vi "Thevenin Source Calibration.vi"(11 "State":T2) -> ()   [LabVIEW 2015]
uses:
  Utility VIs/Type Defs/Speaker ring.ctl
  Cochlear Function Test Suite/LV Source/CFTS Main Panel SubVIs/CFTS-Experiment State.ctl
  Utility VIs/Controls/KListboxEx/KListboxEx.xctl
  Typedefs/Thev-State.ctl
  Typedefs/Thev-Procedure Phase.ctl
  Typedefs/Thev-Progress Table Element.ctl
  Typedefs/Thev-Optimization Result.ctl
  Typedefs/Thev-Parameters.ctl
  Typedefs/Thev-Stimulus.ctl
  Typedefs/Thev-Find.ctl
  Misc VIs/Equipment Control/ER10X/ER10X-Probe.ctl
  Typedefs/Thev-Optimization Parameters.ctl
  D:/Experiment VIs/Misc VIs/Equipment Control/ER10X/ER10XConnect.NET.dll
  Misc VIs/Equipment Control/ER10X/ER10XConnect.NET.dll
  Utility VIs/Conversion VIs/Create Waveform Cluster (2D).vi
  Utility VIs/Math VIs/FFT x(t) to dB,Degrees (2D).vi
panel:
  in  "Test":enum16{"Lengths", "Frequencies"}(ring)
  in  "Nulls":i32(xcontrol) caption="Null frequencies (Hz)"
  out "Probe B":bool
  out "Probe A":bool
  in  "Start":bool
  in  "Stop":bool
  in  "Find":T1={"precision"=10.0, "Nattempts"=6, "Navgs/att"=64} caption="Optimize positions"
  in  "Averages":i32=128
  in  "Speaker":T3
  in  "mic gain":dbl caption="Gain (dB)" min=0.0 max=40.0 step=1.0
  in  "Stimulus":T4={"Resolution (Hz)"=50.0, "Attenuation (dB)"=30.0, "Sampling rate (Hz)"=100000.0}
  out "Stimulus graph":cluster{i32, dbl, dbl[]}(graph)={0, 0.01, []}
  in  "Diameter":dbl=128.0 caption="Cavity diameter (cm)"
  in  "Compute":bool
  out "Log":string
  out "Progress":string[][](table)
  in  "Tabs":T5(tab)
  out "Mic signals":cluster{"offset":dbl, "dx":dbl, "Y":dbl[][]}(graph)
  out "Mic mag":cluster{"offset":dbl, "dx":dbl, "Y":dbl[][]}(graph)
  out "Acquired":i32=256
  out "Magnitude":cluster{"Frequency":dbl[], "Frequency":dbl[]}[](graph)
  out "Phase":cluster{"Frequency":dbl[], "Frequency":dbl[]}[](graph)
  out "Zx mag":cluster{"Frequency":dbl[], "Frequency":dbl[]}[](graph)
  out "Zx phase":cluster{"Frequency":dbl[], "Frequency":dbl[]}[](graph)
  out "Z0":cluster{"Frequency":dbl[], "Frequency":dbl[]}[](graph)
  out "P0":cluster{"Frequency":dbl[], "Frequency":dbl[]}[](graph)
  in  "result":cluster{"Path":path, "error ":errorcluster}
  out "Mic phase":cluster{"offset":dbl, "dx":dbl, "Y":dbl[][]}(graph)
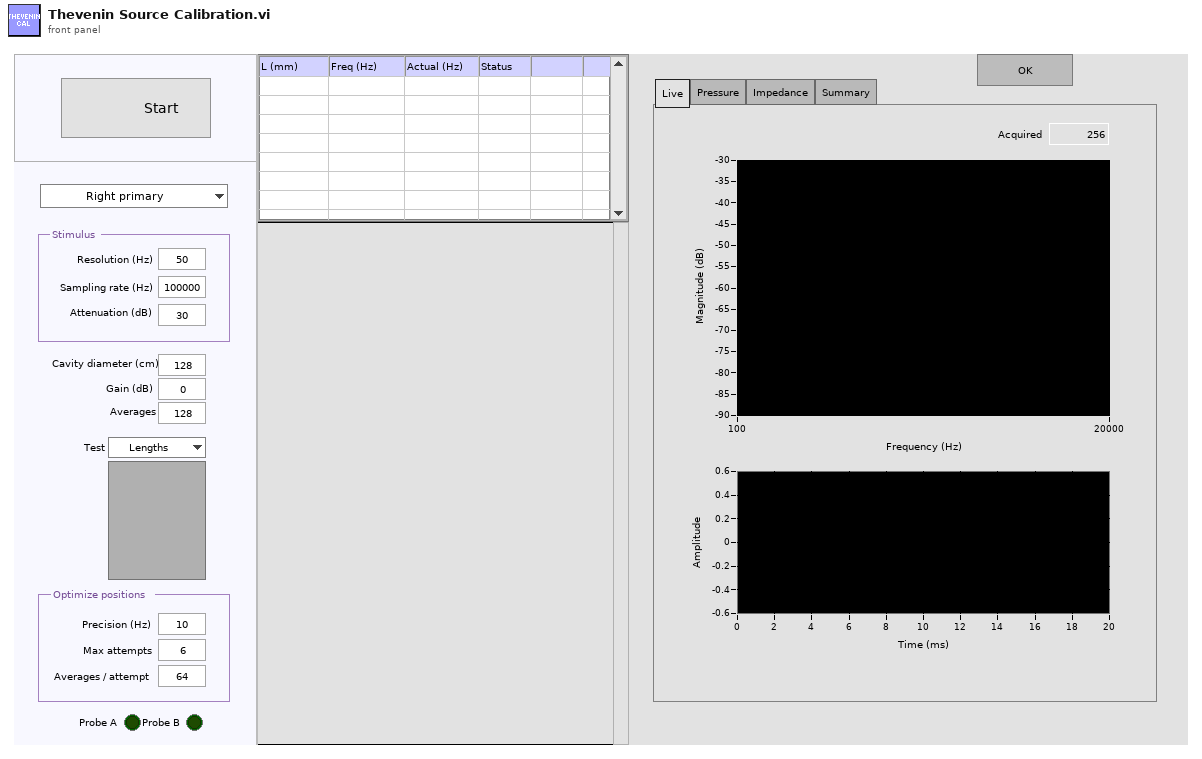
[diagram p1: front panel]
types:
  T1 = cluster{"precision":dbl, "Nattempts":i32, "Navgs/att":i32}
  T2 = typedef "CFTS-Experiment State.ctl" = cluster{"Experimenter":string, "Number":u32, "Right":string, "Left":string, "Data Folder":path, "State File":path, "Version Info":string, "End Exposure Time":dbl, "Exposure Duration":string, "Run #":cluster{"CAP":i16, "ABR":i16, "DP":i16, "VsEP":i16, "MeasSeq":i16, "SubSeq":i16, "SFOAE":i16}}
  T3 = typedef "Speaker ring.ctl" = enum16{"Right primary", "Right secondary", "Left primary", "Left secondary"}
  T4 = cluster{"Resolution (Hz)":dbl, "Attenuation (dB)":dbl, "Sampling rate (Hz)":dbl}
  T5 = enum32{"Live", "Pressure", "Impedance", "Summary"}
  T6 = typedef "Thev-Parameters.ctl" = cluster{"Speaker":enum16{"Right primary", "Right secondary", "Left primary", "Left secondary"}, "Chirp":T7, "Find":T8, "Gain (dB)":dbl, "Navgs":i32, "Diameter":dbl, "test points":dbl[], "Rprobe":T9, "LProbe":T9, "Mode":enum16{"Length", "Freq"}, "Optim":T10}
  T7 = typedef "Thev-Stimulus.ctl" = cluster{"resol (Hz)":dbl, "atten (dB)":dbl, "Fs (Hz)":dbl}
  T8 = typedef "Thev-Find.ctl" = cluster{"precision":dbl, "Nattempts":i32, "Navgs/att":i32}
  T9 = typedef "ER10X-Probe.ctl" = i32
  T10 = typedef "Thev-Optimization Parameters.ctl" = cluster{"Fmin":dbl, "Fmax":dbl}
  T11 = typedef "Thev-State.ctl" = cluster{"next":i32, "ER10X":refnum<k24>, "phase":T12, "progress":T13[], "folder":path, "log":string, "history":cluster{"L":dbl[], "F":dbl[]}, "optim":T14}
  T12 = typedef "Thev-Procedure Phase.ctl" = enum16{"Optimize", "Measure", "Compute", "Finished"}
  T13 = typedef "Thev-Progress Table Element.ctl" = cluster{"Freq":dbl, "Actual":dbl, "Pos":dbl, "Status":enum16{"None", "Measuring", "Finished"}, "Attempts":i32}
  T14 = typedef "Thev-Optimization Result.ctl" = cluster{"MSE":dbl, "Niter":i32, "Linit":dbl[], "Lfinal":dbl[]}
  T15 = typedef "KListboxEx.xctl/Events.ctl" = cluster{"Items Changed":refnum<user-event>, "List Changed":refnum<user-event>}
  T16 = enum16{"Right primary", "Right secondary", "Left primary", "Left secondary"}
  T17 = enum8{"Enabled", "Disabled", "Disabled and Grayed Out"}
  T18 = typedef "Cal Stimulus.ctl" = cluster{"Min Freq (Hz)":dbl, "Max Freq (Hz)":dbl, "Freq Step (Hz)":dbl, "Waveform":enum16{"Chirp", "Weighted"}, "Attenuation (dB)":dbl, "Sample Rate (Hz)":dbl}
  T19 = cluster{"new file path":path, "error out":errorcluster}
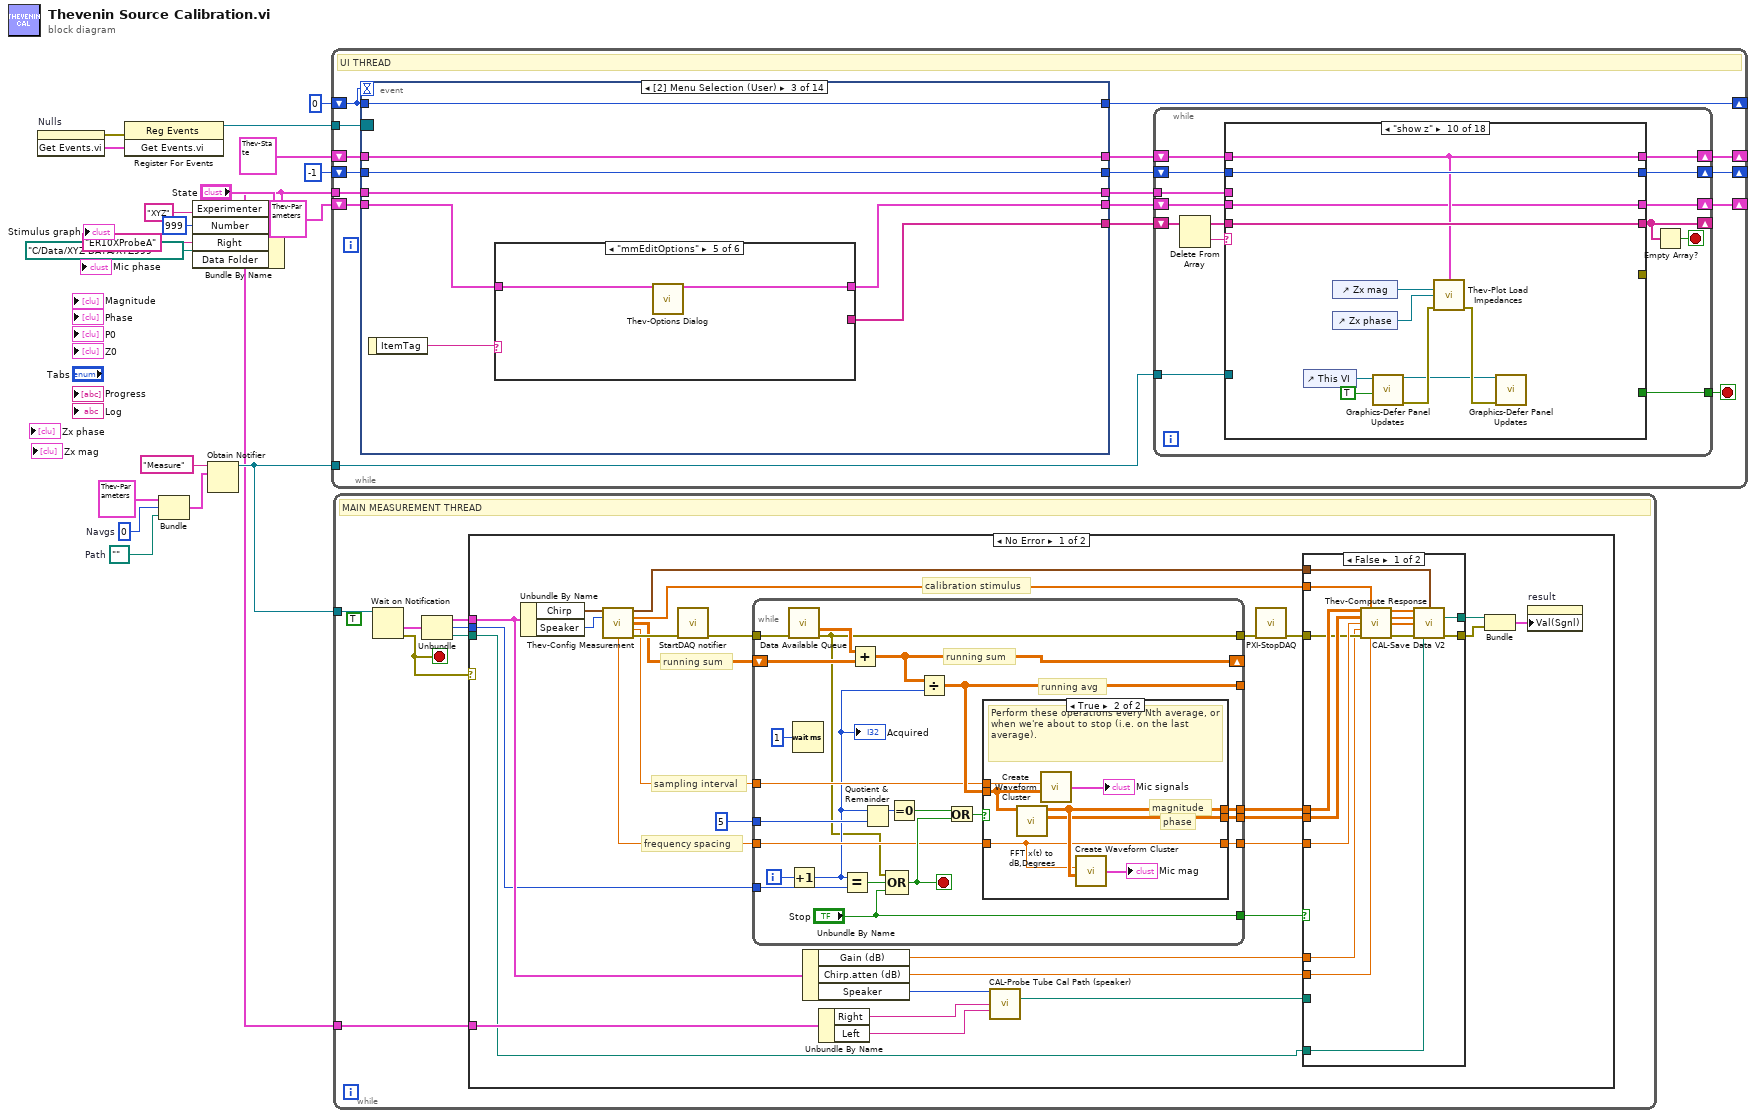
[diagram p0: block diagram]
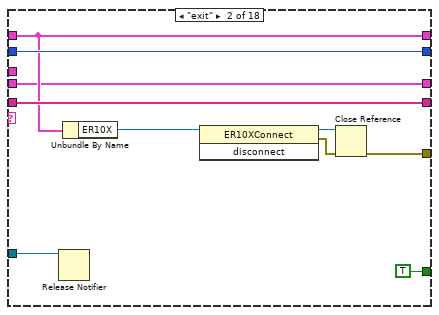
[diagram p6: hidden frame]
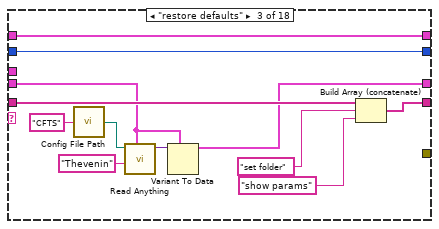
[diagram p7: hidden frame]
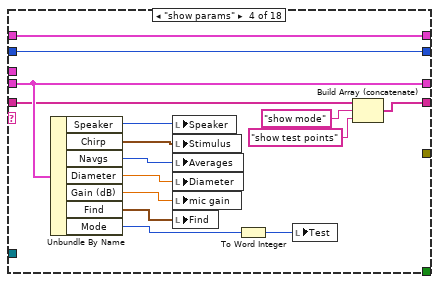
[diagram p8: hidden frame]
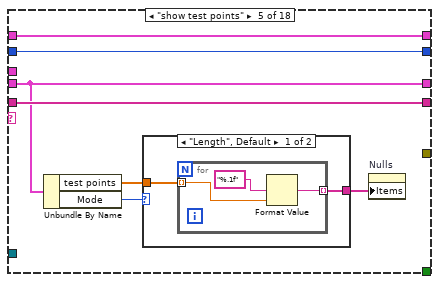
[diagram p9: hidden frame]
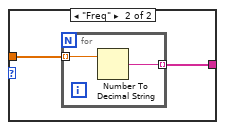
[diagram p10: hidden frame]
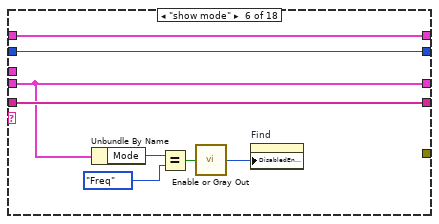
[diagram p11: hidden frame]
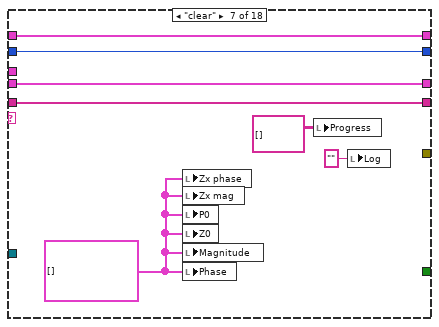
[diagram p12: hidden frame]
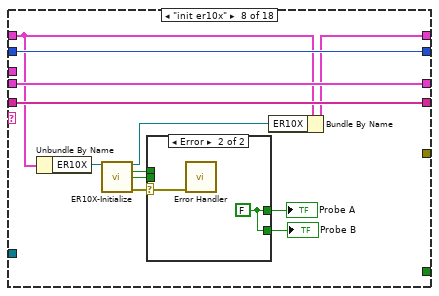
[diagram p13: hidden frame]
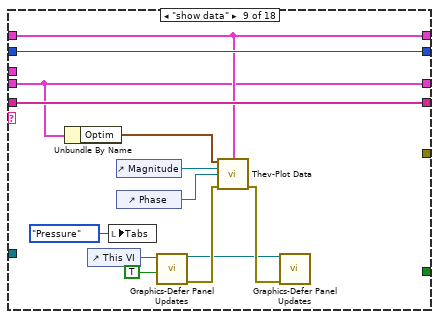
[diagram p15: hidden frame]
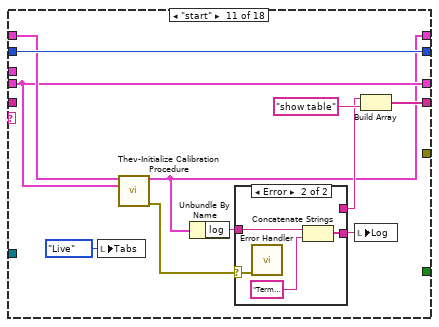
[diagram p16: hidden frame]
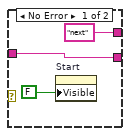
[diagram p17: hidden frame]
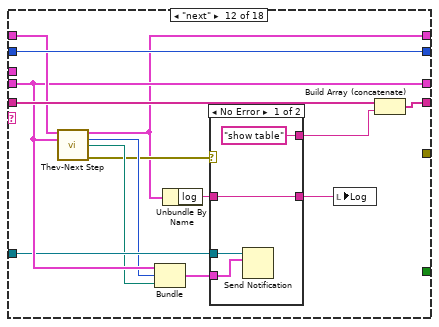
[diagram p18: hidden frame]
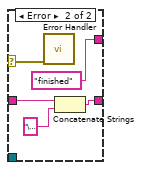
[diagram p19: hidden frame]
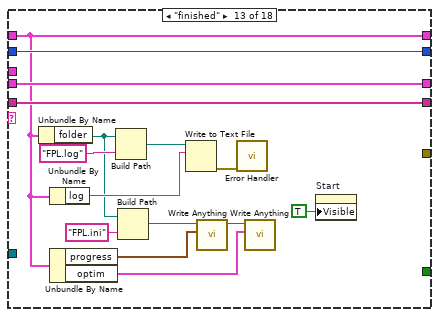
[diagram p20: hidden frame]
diagram:
  w10 = 0  # Navgs
  w9 = path ""  # Path
  n1 = invoke on="Nulls" class="KListboxEx (strict)" method="Get Events.vi"() -> (error out=w8:errorcluster, "Get Events.vi"=w7:T15)  [unwired: 3 in, 1 out]
  n2 = register-events(error in=w8, w7) -> (reference out=w6:refnum<event-registration>)  [unwired: 1 in, 1 out]
  n3 = Bundle("Params"=T6 {"Speaker"=enum."Right primary", "Chirp"={"resol (Hz)"=50.0, "atten (dB)"=20.0, "Fs (Hz)"=100000.0}, "Find"={"precision"=10.0, "Nattempts"=6, "Navgs/att"=64}, "Gain (dB)"=40.0, "Navgs"=128, "Diameter"=0.8, "test points"=[2878.0, 3289.0, 4112.0, 4638.0, 5345.0, 7401.0], "Rprobe"=0, "LProbe"=0, "Mode"=enum."Length", "Optim"={"Fmin"=0.0, "Fmax"=0.0}}, "Navgs"=w10, "Path"=w9) -> (w11:cluster{"Params":T6, "Navgs":i32, "Path":path})  [unwired: 1 in]
  n4 = Bundle By Name(cluster="State", "Experimenter"="XYZ", "Number"=u32 999, "Right"="ER10XProbeA", "Data Folder"=path "C:/Data/XYZ DATA/XYZ999") -> (w5:T2)
  n5 = Obtain Notifier(name (unnamed)="Measure", notification data type=w11) -> (notifier out=w19:refnum<notifier>)  [unwired: 2 in, 2 out]
  n6 = while {
    tunnel: w19 -> [w25]
    shift-right: [w34] -> _
    shift-left: 0 -> [w35]
    shift-right: [w28] -> _
    shift-left: -1 -> [w36]
    tunnel: w5 -> [w33]
    shift-right: [w29] -> _
    shift-left: T6 {"Speaker"=enum."Right primary", "Chirp"={"resol (Hz)"=50.0, "atten (dB)"=20.0, "Fs (Hz)"=100000.0}, "Find"={"precision"=10.0, "Nattempts"=6, "Navgs/att"=64}, "Gain (dB)"=40.0, "Navgs"=128, "Diameter"=0.8, "test points"=[2878.0, 3289.0, 4112.0, 4638.0, 5345.0, 7401.0], "Rprobe"=1, "LProbe"=0, "Mode"=enum."Freq", "Optim"={"Fmin"=500.0, "Fmax"=10000.0}} ("Params") -> [w32]
    shift-right: [w21] -> _
    shift-left: T11 {"next"=0, "ER10X"=refnum, "phase"=enum."Optimize", "progress"=[], "folder"=path "", "log"="", "history"={"L"=[], "F"=[]}, "optim"={"MSE"=0.0, "Niter"=0, "Linit"=[], "Lfinal"=[]}} -> [w23]
    tunnel: w6 -> [w20]
    stop <- w26 stop-if-true
    # "UI THREAD"
    n7 = event shown="[2] Menu Selection (User)" {
      selector: w20 -> [_ _ _ _ _ _ _ _ _ _ _ _ _ _]
      dyn-events: _ -> [_ _ _ _ _ _ _ _ _ _ _ _ _ _]
      timeout: w35 -> [_ _ _ _ _ _ _ _ _ _ _ _ _ _]
      tunnel: w36 -> [w313 w322 w331 w353 w368 w375 w382 w394 w401 w414 w443 w455 w467 w504]
      tunnel: [w313 w322 w331 w353 w368 w375 w382 w394 w401 w414 w443 w455 w467 w504] -> w31
      tunnel: w35 -> [_ w321 w330 w352 w367 w380 w387 w393 w400 w413 w442 w454 w466 w503]
      tunnel: [-1 w321 w330 w352 w367 w380 w387 w393 w400 w413 w442 w454 w466 w503] -> w34
      tunnel: w33 -> [w305 w318 w325 w351 w357 w378 w385 w390 w397 w412 w440 w451 w465 w501]
      tunnel: w32 -> [w303 w320 w328 w350 w366 w379 w386 w392 w399 w403 w441 w453 w461 w502]
      tunnel: [w303 w320 w327 w350 w365 w377 w384 w391 w398 w410 w438 w452 w461 w502] -> w30
      tunnel: [string[] ["init er10x", "restore defaults"] string[] ["exit"] w326 string[] ["start"] w354 _ _ _ _ string[] ["show mode", "show test points"] _ _ w459 string[] ["compute"]] -> w27
      tunnel: [w305 w318 w325 w351 w357 w378 w385 w390 w397 w412 w440 w451 w465 w501] -> w24
      tunnel: w23 -> [w302 w317 w324 w349 w356 w374 w381 w388 w396 w411 w439 w450 w462 w500]
      tunnel: [w302 w317 w324 w349 w355 w374 w381 w388 w396 w411 w439 w450 w457 w500] -> w22
      event Timeout {
        n8 = event-data() -> ()  [unwired: 1 in, 1 out]
        n9 = property on="Nulls" class="KListboxEx (strict)"() -> ("Ref"=w310:refnum<vi>)  [unwired: 2 in, 2 out]
        n10 = property class="LstBox (strict)"(reference=w310, "Horizontal Lines Visible"=TRUE ("Visible Items:Horizontal Lines Visible"), "Allow Item Drag"=FALSE ("Drag/Drop:Allow Dragging")) -> (reference out=w307:refnum<vi>)  [unwired: 1 in, 1 out]
        n11 = for {
          N: 10 -> [_]
          tunnel: w307 -> [w316]
          i -> [w315]
          n12 = property class="LstBox (strict)"(reference=w316, "Active Row"=w315, "Justify"=enum16{"Left", "Center", "Right"}."Center" ("Active Row:Cell Justification")) -> ()  [unwired: 1 in, 2 out]
        }
        n13 = property on="Start" class="Bool"("Visible"=TRUE) -> ()  [unwired: 2 in, 2 out]
      }
      event Panel Close? {
        n14 = event-data() -> ()  [unwired: 1 in, 1 out]
        n15 = event-data("Discard?"=TRUE) -> ()  [unwired: 1 in, 1 out]
      }
      event Menu Selection (User) {
        n16 = event-data() -> ("ItemTag"=w329:string)  [unwired: 1 in]
        n17 = case shown="\"mmEditOptions\"" w329 {
          tunnel: w328 -> [w332 w334 w337 w343 w345 w346]
          tunnel: [w332 w334 w337 w343 w344 w346] -> w327
          tunnel: [_ string[] ["restore defaults"] _ string[] ["exit"] _ string[] ["init er10x"]] -> w326
          frame "", Default {
          }
          frame "mmFileRestore" {
          }
          frame "mmFileSave" {
            n18 = call "Config File Path.vi"("AppName"="CFTS") -> ("Default config file name"=w338:path)
            n19 = call "Write Anything.vi"("Section Name (Name of \"Anything\")"="Thevenin" ("Section Name (Name of \"Anything\")"), "Anything"=w337, "Path (dialog)"=w338) -> ("Error Out"=w336:errorcluster)  [unwired: 7 in, 1 out]
            n20 = case shown="Error" w336 {
              selector: w336 -> [_ w341]
              frame No Error {
                n21 = One Button Dialog(message="Defaults saved.") -> ()  [unwired: 1 in, 1 out]
              }
              frame Error {
                n22 = call "Error Handler.vi"("error in (no error)"=w341) -> ()  [unwired: 13 in, 2 out]
              }
            }
          }
          frame "mmFileExit" {
          }
          frame "mmEditOptions" {
            n23 = call "Thev-Options Dialog.vi"("Cluster In"=w345) -> ("Cluster out"=w344:T6)  [unwired: 13 in, 1 out]
          }
          frame "mmHelpReset" {
          }
        }
      }
      event "Start": Value Change {
        n24 = event-data() -> ()  [unwired: 1 in, 1 out]
      }
      event Value Change {
        n25 = event-data() -> ("NewVal"=w358:T3)  [unwired: 1 in]
        n26 = Bundle By Name(cluster=w366, "Speaker"=w358) -> (w365:T6)
        n27 = Unbundle By Name(w357) -> ("Data Folder"=w364:path)
        n28 = call "Convert-Speaker to Tag.vi"("Speaker"=w358) -> ("Tag"=w359:string)
        n29 = Concatenate Strings("FPL_" ("name or relative path"), w359) -> (w360:string)
        n30 = Build Path(base path=w364, name or relative path=w360) -> (appended path=w362:path)
        n31 = Bundle By Name(cluster=w356, "folder"=w362) -> (w355:T11)
        n32 = call "FileIO-File or Folder Exists.vi"("path"=w362) -> ("Exists?"=w361:bool)  [unwired: 7 in, 3 out]
        n33 = case shown="True" w361 {
          tunnel: [w369 w372] -> w354
          frame False {
            n34 = Build Array("summary" ("String"), "clear" ("String")) -> (w369:string[])
          }
          frame True {
            n35 = Build Array("restore folder" ("String")) -> (w372:string[])
          }
        }
      }
      event "Stimulus": Value Change {
        n36 = event-data() -> ()  [unwired: 1 in, 1 out]
        n37 = Bundle By Name(cluster=w379, "Chirp"="Stimulus") -> (w377:T6)
      }
      event "Diameter": Value Change {
        n38 = event-data() -> ()  [unwired: 1 in, 1 out]
        n39 = Bundle By Name(cluster=w386, "Diameter"="Diameter") -> (w384:T6)
      }
      event "mic gain": Value Change {
        n40 = event-data() -> ()  [unwired: 1 in, 1 out]
        n41 = Bundle By Name(cluster=w392, "Gain (dB)"="mic gain") -> (w391:T6)
      }
      event "Averages": Value Change {
        n42 = event-data() -> ()  [unwired: 1 in, 1 out]
        n43 = Bundle By Name(cluster=w399, "Navgs"="Averages") -> (w398:T6)
      }
      event "Test": Value Change {
        n44 = event-data() -> ("OldVal"=w406:enum16{"Lengths", "Frequencies"}, "NewVal"=w404:enum16{"Lengths", "Frequencies"})  [unwired: 1 in]
        n45 = Not Equal?(x=w406, y=w404) -> (x != y?=w405:bool)
        n46 = case shown="True" w405 {
          tunnel: w404 -> [_ w419]
          tunnel: w403 -> [w415 w418]
          tunnel: [w415 w416] -> w402
          frame False {
          }
          frame True {
            n47 = Unbundle By Name(w418) -> ("test points"=w420:dbl[])
            n48 = for {
              tunnel: w420 -> [w423] mode=indexing
              tunnel: w419 -> [w422]
              tunnel: [w421] -> w417 mode=indexing
              n49 = case shown="\"Lengths\", Default" w422 {
                tunnel: w423 -> [w428 w430]
                tunnel: [w424 w429] -> w421
                frame "Lengths", Default {
                  n50 = Multiply(x=w428, y=4.0) -> (x*y=w426:dbl)
                  n51 = Divide(x=343000.0, y=w426) -> (x/y=w424:dbl)
                }
                frame "Frequencies" {
                  n52 = Multiply(x=w430, y=4.0) -> (x*y=w432:dbl)
                  n53 = Divide(x=343000.0, y=w432) -> (x/y=w429:dbl)
                }
              }
            }
            n54 = Bundle By Name(cluster=w418, "test points"=w417) -> (w416:T6)
          }
        }
        n55 = To Word Integer(number="Test") -> (16bit integer=w408:i16)
        n56 = Bundle By Name(cluster=w402, "Mode"=w408) -> (w410:T6)
      }
      event User Event {
        n57 = event-data() -> ()  [unwired: 1 in, 1 out]
        n58 = property on="Nulls" class="KListboxEx (strict)"() -> ("Items"=w436:string[])  [unwired: 2 in, 2 out]
        n59 = for {
          tunnel: w436 -> [w448] mode=indexing
          tunnel: [w447] -> w437 mode=indexing if=w446
          n60 = Decimal String To Number(string=w448) -> (number=w447:i32)  [unwired: 2 in, 1 out]
          n61 = Greater Than 0?(x=w447) -> (x > 0?=w446:bool)
        }
        n62 = Sort 1D Array(array=w437) -> (sorted array=w435:i32[])
        n63 = for {
          tunnel: w435 -> [w445] mode=indexing
          tunnel: [w444] -> w434 mode=indexing
          n64 = Number To Decimal String(number=w445) -> (decimal integer string=w444:string)  [unwired: 1 in]
        }
        n65 = Bundle By Name(cluster=w441, "test points"=w435) -> (w438:T6)
        n66 = property on="Nulls" class="KListboxEx (strict)"("Items"=w434) -> ()  [unwired: 2 in, 2 out]
      }
      event "Find": Value Change {
        n67 = event-data() -> ()  [unwired: 1 in, 1 out]
        n68 = Bundle By Name(cluster=w453, "Find"="Find") -> (w452:T6)
      }
      event "result": Value Change {
        n69 = event-data() -> ("NewVal.Path"=w463:path, "NewVal.error"=w464:errorcluster)  [unwired: 1 in]
        n70 = case shown="No Error" w464 {
          selector: w464 -> [_ w492]
          tunnel: w463 -> [w470 _]
          tunnel: w462 -> [w472 w497]
          tunnel: [w473 w494] -> w457
          tunnel: w461 -> [w471 _]
          tunnel: [w468 w491] -> w460
          frame No Error {
            n71 = Empty String/Path?(string/path=w470) -> (empty?=w469:bool)
            n72 = case shown="False" w469 {
              tunnel: [w476 w486] -> w473
              tunnel: w472 -> [w480 w490]
              tunnel: w471 -> [w479 _]
              tunnel: w470 -> [w477 _]
              tunnel: [w474 w484] -> w468
              frame False {
                n73 = call "Thev-Process Response.vi"("State in"=w480, "Params"=w479, "Path"=w477) -> ("State out"=w476:T11, "error out"=w478:errorcluster)  [unwired: 11 in]
                n74 = call "Error Handler.vi"("error in (no error)"=w478) -> ()  [unwired: 13 in, 2 out]
                n75 = Unbundle By Name(w476) -> ("phase"=w475:T12)
                n76 = case shown="\"Compute\"" w475 {
                  tunnel: [w481 string[] ["compute", "show data"]] -> w474
                  frame "Optimize", Default {
                    n77 = Build Array("next") -> (w481:string[])
                  }
                  frame "Compute" {
                  }
                }
              }
              frame True {
                n78 = Unbundle By Name(w490) -> ("log"=w489:string)
                n79 = Concatenate Strings(w489, "\nAborted.") -> (w485:string)
                n80 = Bundle By Name(cluster=w490, "log"=w485) -> (w486:T11)
                n81 = Build Array("finished" ("String")) -> (w484:string[])
              }
            }
          }
          frame Error {
            n82 = call "Error Handler.vi"("error in (no error)"=w492) -> ()  [unwired: 13 in, 2 out]
            n83 = Unbundle By Name(w497) -> ("log"=w496:string)
            n84 = Concatenate Strings(w496, "Terminated with error.") -> (w493:string)
            n85 = Bundle By Name(cluster=w497, "log"=w493) -> (w494:T11)
            n86 = Build Array("finished" ("String")) -> (w491:string[])
          }
        }
        n87 = Unbundle By Name(w457) -> ("log"=w456:string)
        n88 = local write "Log"(w456) -> ()
        n89 = Build Array (concatenate)(w460, "show table" ("element")) -> (w459:string[])
      }
      event "Compute": Value Change {
        n90 = event-data() -> ()  [unwired: 1 in, 1 out]
      }
    }
    n91 = while {
      shift-right: [w48] -> w29
      shift-left: w30 -> [w49]
      shift-right: [w47] -> w28
      shift-left: w31 -> [w50]
      shift-right: [w43] -> _
      shift-left: w27 -> [w45]
      tunnel: w25 -> [w41]
      tunnel: [w40] -> w26
      tunnel: w24 -> [w39]
      shift-right: [w38] -> w21
      shift-left: w22 -> [w37]
      stop <- w42 stop-if-true
      n92 = Delete From Array(array=w45) -> (deleted portion=w44:string, array with subset deleted=w46:string[])  [unwired: 2 in]
      n93 = case shown="\"show z\"" w44 {
        tunnel: w50 -> [w54 w64 w76 w91 w98 w115 w122 w134 w151 w162 w173 w194 w218 w240 w257 w263 w284 w301]
        tunnel: [w54 w64 w76 w91 w98 w115 w122 w134 w151 w162 w173 w194 w218 w240 w257 w263 w284 w301] -> w47
        tunnel: w49 -> [w53 w58 w72 w90 w95 w112 w121 w133 w141 w152 w171 w191 w217 w239 w249 w262 w278 w300]
        tunnel: [w53 w58 w71 w90 w95 w112 w121 w133 w141 w152 w171 w191 w217 w239 w249 w262 w278 w300] -> w48
        tunnel: w46 -> [w52 w63 w75 w84 w97 w114 w120 w132 w150 w161 _ w193 w216 w238 w256 w261 w272 w299]
        tunnel: [w52 w63 w70 w81 w97 w114 w120 w132 w150 w161 w168 w185 w216 w229 w245 w261 w283 w299] -> w43
        tunnel: w41 -> [_ w62 _ _ _ _ _ _ _ _ _ w190 _ _ _ _ _ _]
        tunnel: [_ TRUE _ _ _ _ _ _ _ _ _ _ _ _ _ _ _ _] -> w40
        tunnel: w39 -> [_ _ _ _ _ _ _ _ _ _ _ _ _ _ w248 _ w271 w297]
        tunnel: [w51 w60 w67 w86 w96 w113 w119 w131 w148 w159 w165 w183 w207 w231 w246 w260 w279 w298] -> w38
        tunnel: w37 -> [w51 w60 w67 w86 w96 w113 w119 w124 w148 w159 w172 w192 w207 w223 w247 w260 w282 w298]
        tunnel: [_ w59 _ _ _ _ _ _ _ _ _ _ _ _ _ _ _ _] -> _
        frame "", Default {
        }
        frame "exit" {
          n94 = Release Notifier(notifier=w62) -> ()  [unwired: 2 in, 3 out]
          n95 = Unbundle By Name(w60) -> ("ER10X"=w55:refnum<k24>)
          n96 = invoke class="ER10XConnect" method="disconnect"(reference=w55) -> (reference out=w56:refnum<k24>, error out=w57:errorcluster)  [unwired: 2 in, 1 out]
          n97 = Close Reference(reference=w56, error in (no error)=w57) -> (error out=w59:errorcluster)
        }
        frame "restore defaults" {
          n98 = call "Config File Path.vi"("AppName"="CFTS") -> ("Default config file name"=w68:path)
          n99 = call "Read Anything.vi"("Type of Anything"=w72, "Section Name (Name of \"Type of Anything\")"="Thevenin" ("Section Name (Name of \"Type of Anything\")"), "Path (dialog)"=w68) -> ("Anything"=w73:variant)  [unwired: 6 in, 2 out]
          n100 = Variant To Data(type=w72, Variant=w73) -> (data=w71:T6)  [unwired: 1 in, 1 out]
          n101 = Build Array (concatenate)(w75, "set folder", "show params") -> (w70:string[])
        }
        frame "show params" {
          n102 = Unbundle By Name(w90) -> ("Speaker"=w89:T16, "Chirp"=w88:T7, "Navgs"=w87:i32, "Diameter"=w85:dbl, "Gain (dB)"=w83:dbl, "Find"=w82:T8, "Mode"=w79:enum16{"Length", "Freq"})
          n103 = local write "Speaker"(w89) -> ()
          n104 = local write "Stimulus"(w88) -> ()
          n105 = local write "Averages"(w87) -> ()
          n106 = local write "Diameter"(w85) -> ()
          n107 = local write "mic gain"(w83) -> ()
          n108 = local write "Find"(w82) -> ()
          n109 = To Word Integer(number=w79) -> (16bit integer=w78:i16)
          n110 = local write "Test"(w78) -> ()
          n111 = Build Array (concatenate)(w84, "show mode", "show test points" ("element")) -> (w81:string[])
        }
        frame "show test points" {
          n112 = Unbundle By Name(w95) -> ("test points"=w94:dbl[], "Mode"=w93:enum16{"Length", "Freq"})
          n113 = case shown="\"Length\", Default" w93 {
            tunnel: w94 -> [w99 w104]
            tunnel: [w100 w105] -> w92
            frame "Length", Default {
              n114 = for {
                tunnel: [w103] -> w100 mode=indexing
                tunnel: w99 -> [w102] mode=indexing
                n115 = Format Value(format string="%.1f" ("string (\"\")"), value (0)=w102) -> (output string=w103:string)  [unwired: 1 in]
              }
            }
            frame "Freq" {
              n116 = for {
                tunnel: [w107] -> w105 mode=indexing
                tunnel: w104 -> [w106] mode=indexing
                n117 = Number To Decimal String(number=w106) -> (decimal integer string=w107:string)  [unwired: 1 in]
              }
            }
          }
          n118 = property on="Nulls" class="KListboxEx (strict)"("Items"=w92) -> ()  [unwired: 2 in, 2 out]
        }
        frame "show mode" {
          n119 = Unbundle By Name(w112) -> ("Mode"=w111:enum16{"Length", "Freq"})
          n120 = Equal?(x=w111, y=enum16{"Length", "Freq"}."Freq") -> (x = y?=w109:bool)
          n121 = call "Enable or Gray Out.vi"("Boolean"=w109) -> ("Disabled"=w108:T17)
          n122 = property on="Find" class="Clust (strict)"("DisabledEnum"=w108) -> ()  [unwired: 2 in, 2 out]
        }
        frame "clear" {
          w116 = cluster{"Frequency":dbl[], "Frequency":dbl[]}[] [] ("Magnitude")
          n123 = local write "Zx phase"(w116) -> ()
          n124 = local write "Zx mag"(w116) -> ()
          n125 = local write "P0"(w116) -> ()
          n126 = local write "Z0"(w116) -> ()
          n127 = local write "Magnitude"(w116) -> ()
          n128 = local write "Phase"(w116) -> ()
          n129 = local write "Progress"(string[][] [] ("Progress")) -> ()
          n130 = local write "Log"("" ("Log")) -> ()
        }
        frame "init er10x" {
          n131 = Unbundle By Name(w124) -> ("ER10X"=w123:refnum<k24>)
          n132 = call "ER10X-Initialize.vi"("ER10X"=w123) -> (".NET reference"=w130:refnum<k24>, "ProbeA"=w128:bool, "ProbeB"=w127:bool, "error out"=w129:errorcluster)  [unwired: 11 in]
          n133 = case shown="Error" w129 {
            selector: w129 -> [_ w138]
            tunnel: [w135 w137] -> w126
            tunnel: [w136 w137] -> w125
            tunnel: w128 -> [w135 _]
            tunnel: w127 -> [w136 _]
            frame No Error {
            }
            frame Error {
              w137 = FALSE
              n134 = call "Error Handler.vi"("error in (no error)"=w138) -> ()  [unwired: 13 in, 2 out]
            }
          }
          "Probe A" <- w126
          "Probe B" <- w125
          n135 = Bundle By Name(cluster=w124, "ER10X"=w130) -> (w131:T11)
        }
        frame "show data" {
          n136 = Unbundle By Name(w141) -> ("Optim"=w140:T10)
          n137 = control-ref of="This VI"() -> (w146:refnum<vi>)
          n138 = local write "Tabs"(T5."Pressure" ("Tabs")) -> ()
          n139 = control-ref of="Magnitude"() -> (w149:refnum<vi>)
          n140 = control-ref of="Phase"() -> (w147:refnum<vi>)
          n141 = call "Graphics-Defer Panel Updates.vi"("VI"=w146, "Defer (F)"=TRUE) -> ("VI out"=w142:refnum<vi>, "error out"=w144:errorcluster)  [unwired: 12 in]
          n142 = call "Thev-Plot Data.vi"("Optim"=w140, "State"=w148, "Mag graph"=w149, "Phase graph"=w147, "error in (no error)"=w144) -> ("error out"=w143:errorcluster)  [unwired: 10 in]
          n143 = call "Graphics-Defer Panel Updates.vi"("VI"=w142, "error in (no error)"=w143) -> ()  [unwired: 12 in, 2 out]
        }
        frame "show z" {
          n144 = control-ref of="This VI"() -> (w157:refnum<vi>)
          n145 = control-ref of="Zx mag"() -> (w160:refnum<vi>)
          n146 = control-ref of="Zx phase"() -> (w158:refnum<vi>)
          n147 = call "Graphics-Defer Panel Updates.vi"("VI"=w157, "Defer (F)"=TRUE) -> ("VI out"=w153:refnum<vi>, "error out"=w155:errorcluster)  [unwired: 12 in]
          n148 = call "Thev-Plot Load Impedances.vi"("State"=w159, "Mag graph"=w160, "Phase graph"=w158, "error in (no error)"=w155) -> ("error out"=w154:errorcluster)  [unwired: 11 in]
          n149 = call "Graphics-Defer Panel Updates.vi"("VI"=w153, "error in (no error)"=w154) -> ()  [unwired: 12 in, 2 out]
        }
        frame "start" {
          n150 = local write "Tabs"(T5."Live" ("Tabs")) -> ()
          n151 = call "Thev-Initialize Calibration Procedure.vi"("State in"=w172, "Params"=w171) -> ("State out"=w165:T11, "error out"=w170:errorcluster)  [unwired: 12 in]
          n152 = Unbundle By Name(w165) -> ("log"=w164:string)
          n153 = case shown="Error" w170 {
            selector: w170 -> [_ w180]
            tunnel: w164 -> [w175 w178]
            tunnel: [w175 w179] -> w169
            tunnel: ["next" ("String") _] -> w166
            frame No Error {
              n154 = property on="Start" class="Bool"("Visible"=FALSE) -> ()  [unwired: 2 in, 2 out]
            }
            frame Error {
              n155 = call "Error Handler.vi"("error in (no error)"=w180) -> ()  [unwired: 13 in, 2 out]
              n156 = Concatenate Strings(w178, "Terminated with error." ("Log")) -> (w179:string)
            }
          }
          n157 = local write "Log"(w169) -> ()
          n158 = Build Array(w166, "show table") -> (w168:string[])
        }
        frame "next" {
          n159 = call "Thev-Next Step.vi"("State in"=w192, "Params"=w191) -> ("State out"=w183:T11, "Navgs"=w189:i32, "Path"=w188:path, "error out"=w186:errorcluster)  [unwired: 10 in]
          n160 = Bundle("Params"=w191, "Navgs"=w189, "Path"=w188) -> (w187:cluster{"Params":T6, "Navgs":i32, "Path":path})  [unwired: 1 in]
          n161 = Unbundle By Name(w183) -> ("log"=w182:string)
          n162 = case shown="No Error" w186 {
            selector: w186 -> [_ w203]
            tunnel: w190 -> [w198 _]
            tunnel: w187 -> [w197 _]
            tunnel: ["show table" "finished"] -> w184
            tunnel: w182 -> [w195 w201]
            tunnel: [w195 w200] -> w181
            frame No Error {
              n163 = Send Notification(notification=w197, notifier=w198) -> ()  [unwired: 1 in, 2 out]
            }
            frame Error {
              n164 = call "Error Handler.vi"("error in (no error)"=w203) -> ()  [unwired: 13 in, 2 out]
              n165 = Concatenate Strings(w201, "\nTerminated with error.") -> (w200:string)
            }
          }
          n166 = local write "Log"(w181) -> ()
          n167 = Build Array (concatenate)(w193, w184) -> (w185:string[])
        }
        frame "finished" {
          n168 = Unbundle By Name(w207) -> ("folder"=w209:path)
          n169 = Unbundle By Name(w207) -> ("log"=w211:string)
          n170 = Unbundle By Name(w207) -> ("progress"=w206:T13[], "optim"=w204:T14)
          n171 = Build Path(base path=w209, name or relative path="FPL.log") -> (appended path=w213:path)
          n172 = Build Path(base path=w209, name or relative path="FPL.ini") -> (appended path=w208:path)
          n173 = Write to Text File(file (use dialog)=w213, text=w211) -> (error out=w212:errorcluster)  [unwired: 2 in, 2 out]
          n174 = call "Write Anything.vi"("Anything"=w206, "Path (dialog)"=w208) -> ("Path out"=w205:path)  [unwired: 8 in, 1 out]
          n175 = call "Error Handler.vi"("error in (no error)"=w212) -> ()  [unwired: 13 in, 2 out]
          n176 = call "Write Anything.vi"("Anything"=w204, "Path (dialog)"=w205) -> ()  [unwired: 8 in, 2 out]
          n177 = property on="Start" class="Bool"("Visible"=TRUE) -> ()  [unwired: 2 in, 2 out]
        }
        frame "restore folder" {
          n178 = Unbundle By Name(w223) -> ("folder"=w235:path)
          n179 = Unbundle By Name(w223) -> ("progress"=w230:T13[])
          n180 = Unbundle By Name(w223) -> ("optim"=w222:T14)
          n181 = Build Path(base path=w235, name or relative path="FPL.ini") -> (appended path=w224:path)
          n182 = Build Path(base path=w235, name or relative path="FPL.log") -> (appended path=w234:path)
          n183 = call "Read Anything.vi"("Type of Anything"=w230, "Path (dialog)"=w224) -> ("Error Out"=w233:errorcluster, "Anything"=w232:variant)  [unwired: 7 in, 1 out]
          n184 = Read from Text File(file (use dialog)=w234) -> (text=w227:string)  [unwired: 3 in, 3 out]
          n185 = Variant To Data(error in=w233, type=w230, Variant=w232) -> (data=w228:T13[], error out=w220:errorcluster)
          n186 = call "Read Anything.vi"("Type of Anything"=w222, "Error In"=w220, "Path (dialog)"=w224) -> ("Error Out"=w226:errorcluster, "Anything"=w225:variant)  [unwired: 6 in, 1 out]
          n187 = Variant To Data(error in=w226, type=w222, Variant=w225) -> (data=w221:T14)  [unwired: 1 out]
          n188 = local write "Log"(w227) -> ()
          n189 = Bundle By Name(cluster=w223, "log"=w227, "progress"=w228, "optim"=w221) -> (w231:T11)
          n190 = Build Array (concatenate)(w238, string[] ["summary", "show z", "show data", "show table"]) -> (w229:string[])
        }
        frame "set folder" {
          n191 = Unbundle By Name(w249) -> ("Speaker"=w253:T16)
          n192 = Unbundle By Name(w248) -> ("Data Folder"=w250:path)
          n193 = call "Convert-Speaker to Tag.vi"("Speaker"=w253) -> ("Tag"=w255:string)
          n194 = Concatenate Strings("FPL_" ("name or relative path"), w255) -> (w254:string)
          n195 = Build Path(base path=w250, name or relative path=w254) -> (appended path=w252:path)
          n196 = call "FileIO-File or Folder Exists.vi"("path"=w252) -> ("Exists?"=w244:bool)  [unwired: 7 in, 3 out]
          n197 = Bundle By Name(cluster=w247, "folder"=w252) -> (w246:T11)
          n198 = Select(t="restore folder" ("String"), s=w244, f="") -> (s? t:f=w242:string)
          n199 = Build Array (concatenate)(w256, w242) -> (w245:string[])
        }
        frame "show table" {
          n200 = Unbundle By Name(w260) -> ("progress"=w258:T13[])
          n201 = control-ref of="Progress"() -> (w259:refnum<vi>)
          n202 = call "Thev-Show Progress Table.vi"("Table in"=w259, "progress"=w258) -> ()  [unwired: 14 in]
        }
        frame "compute" {
          n203 = Unbundle By Name(w278) -> ("Optim"=w277:T10, "Speaker"=w273:T16)
          n204 = Unbundle By Name(w271) -> ("Right"=w275:string, "Left"=w274:string)
          n205 = Unbundle By Name(w282) -> ("folder"=w269:path)
          n206 = Unbundle By Name(w282) -> ("log"=w281:string)
          n207 = call "CAL-Probe Tube Cal Path (speaker).vi"("Speaker"=w273, "Right"=w275, "Left"=w274) -> ("Probe Tube Cal Path"=w270:path, "error out"=w268:errorcluster)  [unwired: 11 in]
          n208 = call "Thev-Compute.vi"("folder"=w269, "Options"=w277, "probe tube path"=w270, "error in (no error)"=w268) -> ("log"=w265:string, "Result"=w267:T14, "error out"=w276:errorcluster)  [unwired: 9 in]
          n209 = Concatenate Strings(w281, "---Compute Thevenin equivalent source---\n", w265) -> (w264:string)
          n210 = case shown="Error" w276 {
            selector: w276 -> [_ w286]
            tunnel: [string[] ["summary", "show z", "finished"] string[] ["finished"]] -> w266
            frame No Error {
            }
            frame Error {
              n211 = call "Error Handler.vi"("error in (no error)"=w286) -> ()  [unwired: 13 in, 2 out]
            }
          }
          n212 = local write "Log"(w264) -> ()
          n213 = Bundle By Name(cluster=w282, "log"=w264, "optim"=w267) -> (w279:T11)
          n214 = Build Array (concatenate)(w272, w266) -> (w283:string[])
        }
        frame "summary" {
          n215 = Unbundle By Name(w297) -> ("Data Folder"=w296:path)
          n216 = control-ref of="This VI"() -> (w292:refnum<vi>)
          n217 = control-ref of="P0"() -> (w295:refnum<vi>)
          n218 = control-ref of="Z0"() -> (w294:refnum<vi>)
          n219 = call "Graphics-Defer Panel Updates.vi"("VI"=w292, "Defer (F)"=TRUE) -> ("VI out"=w290:refnum<vi>, "error out"=w291:errorcluster)  [unwired: 12 in]
          n220 = call "Thev-Show Summary.vi"("Data Folder"=w296, "P0"=w295, "Z0"=w294, "error in (no error)"=w291) -> ("error out"=w289:errorcluster)  [unwired: 11 in]
          n221 = call "Graphics-Defer Panel Updates.vi"("VI"=w290, "error in (no error)"=w289) -> ()  [unwired: 12 in, 2 out]
          n222 = local write "Tabs"(T5."Summary" ("Tabs")) -> ()
        }
      }
      n223 = Empty Array?(array=w43) -> (empty?=w42:bool)
    }
  }
  n224 = while {
    tunnel: w19 -> [w511]
    tunnel: w5 -> [w510]
    stop <- w505 stop-if-true
    (unwired) TRUE
    # "MAIN MEASUREMENT THREAD"
    n225 = Wait on Notification(notifier=w511) -> (notification=w509:cluster{"Params":T6, "Navgs":i32, "Path":path}, error out=w505:errorcluster)  [unwired: 3 in, 2 out]
    n226 = Unbundle(w509) -> ("Params"=w508:T6, "Navgs"=w507:i32, "Path"=w506:path)
    n227 = case shown="No Error" w505 {
      tunnel: w510 -> [w525 _]
      tunnel: w508 -> [w517 _]
      tunnel: w507 -> [w513 _]
      tunnel: w506 -> [w512 _]
      frame No Error {
        # "calibration stimulus"
        # "frequency spacing"
        # "sampling interval"
        # "running sum"
        n228 = Unbundle By Name(w517) -> ("Chirp"=w515:T7, "Speaker"=w524:T16)
        n229 = call "Thev-Config Measurement.vi"("Chirp spec in"=w515, "Speaker"=w524) -> ("Cal Stimulus"=w533:T18, "Stimulus"=w514:dbl[], "Mic Avg"=w539:dbl[][], "dt (ms)"=w537:dbl, "df (Hz)"=w538:dbl, "error out"=w540:errorcluster)  [unwired: 8 in]
        n230 = call "StartDAQ notifier.vi"("error in (no error)"=w540) -> ("error out"=w532:errorcluster)  [unwired: 6 in]
        n231 = while {
          tunnel: w532 -> [w578]
          tunnel: [w558] -> w531
          tunnel: w513 -> [w575]
          shift-right: [w573] -> _
          shift-left: w539 -> [w574]
          tunnel: [w572] -> _
          tunnel: 5 -> [w571]
          tunnel: w538 -> [w566]
          tunnel: [w565] -> w536
          tunnel: [w564] -> w535
          tunnel: w537 -> [w563]
          tunnel: [w562] -> w534
          tunnel: ["Stop"] -> w522
          i -> [w577]
          stop <- w567 stop-if-true
          # "running avg"
          # "running sum"
          n232 = call "Data Available Queue.vi"("error in (no error)"=w578) -> ("AI Waveforms"=w560:dbl[][], "error out"=w558:errorcluster)  [unwired: 10 in, 3 out]
          n233 = Increment(x=w577) -> (x+1=w561:i32)
          "Acquired" <- w561
          n234 = Wait (ms)(milliseconds to wait=u32 1) -> ()  [unwired: 1 out]
          n235 = Equal?(x=w561, y=w575) -> (x = y?=w576:bool)
          n236 = Add(x=w560, y=w574) -> (x+y=w573:dbl[][])
          n237 = Quotient & Remainder(x=w561, y=w571) -> (x-y*floor(x/y)=w570:i32)  [unwired: 1 out]
          n238 = Compound Arithmetic op=OR(w558, w576, "Stop") -> (w567:bool)
          n239 = Equal To 0?(x=w570) -> (x = 0?=w568:bool)
          n240 = Divide(x=w573, y=w561) -> (x/y=w572:dbl[][])
          n241 = Or(x=w568, y=w567) -> (x .or. y?=w569:bool)
          n242 = case shown="True" w569 {
            tunnel: w572 -> [_ w582]
            tunnel: w566 -> [_ w579]
            tunnel: [_ w584] -> w565
            tunnel: [_ w583] -> w564
            tunnel: w563 -> [_ w581]
            tunnel: [_ w579] -> w562
            frame False {
            }
            frame True {
              # "phase"
              # "magnitude"
              # "Perform these operations every Nth average, or when we're about to stop (i.e. on the last average)."
              n243 = call-poly "FFT x(t) to dB,Degrees.vi"("X(t)"=w582) -> ("+Freq Phase of FFT (degrees)"=w583:dbl[][], "+Freq. Mag of FFT (dB rms)"=w584:dbl[][])  [unwired: 9 in]
              n244 = call-poly "Create Waveform Cluster.vi"("dx"=w581, "Array"=w582) -> ("waveform cluster"=→"Mic signals":cluster{"offset":dbl, "dx":dbl, "Y":dbl[][]})  [unwired: 3 in]
              n245 = call-poly "Create Waveform Cluster.vi"("dx"=w579, "Array"=w584) -> ("waveform cluster"=→"Mic mag":cluster{"offset":dbl, "dx":dbl, "Y":dbl[][]})  [unwired: 3 in]
            }
          }
        }
        n246 = Unbundle By Name(w517) -> ("Gain (dB)"=w516:dbl, "Chirp.atten (dB)"=w523:dbl, "Speaker"=w521:T16)
        n247 = Unbundle By Name(w525) -> ("Right"=w529:string, "Left"=w528:string)
        n248 = call "CAL-Probe Tube Cal Path (speaker).vi"("Speaker"=w521, "Right"=w529, "Left"=w528) -> ("Probe Tube Cal Path"=w527:path)  [unwired: 11 in, 1 out]
        n249 = call "PXI-StopDAQ.vi"("error in (no error)"=w531) -> ("error out"=w526:errorcluster)  [unwired: 6 in]
        n250 = case shown="False" w522 {
          tunnel: w536 -> [w555 _]
          tunnel: w535 -> [w554 _]
          tunnel: w534 -> [w553 _]
          tunnel: w533 -> [w541 _]
          tunnel: w527 -> [_ _]
          tunnel: w526 -> [w552 w556]
          tunnel: w514 -> [w542 _]
          tunnel: w512 -> [w551 _]
          tunnel: w523 -> [w550 _]
          tunnel: [w549 w556] -> w519
          tunnel: [w548 _] -> w520
          tunnel: w516 -> [w543 _]
          frame False {
            n251 = call "Thev-Compute Response.vi"("Mag"=w555, "Stimulus"=w542, "Phase"=w554, "df (Hz)"=w553, "Probe Mic Gain (dB)"=w543, "error in (no error)"=w552, "Attenuation (dB)"=w550) -> ("ASTF Mag"=w544:dbl[], "ASTF Phase"=w545:dbl[], "Frequency"=w546:dbl[], "error out"=w547:errorcluster)  [unwired: 5 in]
            n252 = call "CAL-Save Data V2.vi"("Mag"=w544, "Cal Stimulus"=w541, "Phase"=w545, "Frequency"=w546, "error in (no error)"=w547, "path"=w551) -> ("new file path"=w548:path, "error out"=w549:errorcluster)  [unwired: 8 in]
          }
          frame True {
          }
        }
        n253 = Bundle("new file path"=w520, "error out"=w519) -> (w518:T19)  [unwired: 1 in]
        n254 = property on="result" class="Clust (strict)"("Val(Sgnl)"=w518) -> ()  [unwired: 2 in, 2 out]
      }
      frame Error {
      }
    }
  }
